vi "Create Master Instance (Serial).vi"(4 "flow control (None)":u16(ring) items=["None", "XON/XOFF", "RTS/CTS", "XON/XOFF & RTS/CTS", "DTR/DSR", "XON/XOFF & DTR/DSR"], 5 "serial type":enum16{"RTU", "ASCII"}(ring), 6 "parity (Even)":u16(ring)=2 items=["None", "Odd", "Even"], 7 "unit ID":u8=1, 8 "error in (no error)":errorcluster, 10 "baud rate (9600)":u32=9600, 11 "VISA resource name":refnum<visa-resource-name>) -> (0 "error out":errorcluster, 3 "serial master instance":refnum<class "Modbus Master.lvclass">)   [LabVIEW 2015, in "Modbus Master.lvclass"]
doc: "Creates a serial or TCP Modbus master instance. You must manually select the polymorphic instance to use."
uses:
  <vilib>/Modbus/master/Modbus Master.lvclass
  <vilib>/Modbus/subvis/Transmission Data Unit (ADU)/RTU Data Unit/RTU Data Unit.lvclass
  <vilib>/Modbus/subvis/Transmission Data Unit (ADU)/ASCII Data Unit/ASCII Data Unit.lvclass
  <vilib>/Modbus/subvis/Transmission Data Unit (ADU)/Transmission Data Unit/Transmission Data Unit.lvclass/Transmission Data Unit.ctl
  <vilib>/Modbus/subvis/Protocol/Serial/Serial Master/Serial Master.lvclass
  <vilib>/Modbus/subvis/Protocol/Serial/Serial Master/Serial Master.lvclass/Serial Master.ctl
  <vilib>/Modbus/master/Modbus Master.lvclass/Modbus Master.ctl
  <vilib>/Modbus/subvis/Modbus API/Modbus API.lvclass/Modbus API.ctl
  <vilib>/Modbus/subvis/Protocol/Serial/Serial Master/Data Access/Serial Data Unit/Write Serial Data Unit.vi
  <vilib>/Modbus/subvis/Protocol/Serial/Serial Master/Data Access/Baud Rate/Write Baud Rate.vi
  <vilib>/Modbus/subvis/Protocol/Serial/Serial Master/Data Access/Parity/Write Parity.vi
  <vilib>/Modbus/subvis/Protocol/Serial/Serial Master/Data Access/VISA resource name/Write VISA resource name.vi
  <vilib>/Modbus/subvis/Protocol/Serial/Serial Master/Data Access/Flow Control/Write Flow Control.vi
  <vilib>/Modbus/subvis/Modbus API/Modbus API.lvclass
  <vilib>/Modbus/subvis/Transmission Data Unit (ADU)/Transmission Data Unit/Transmission Data Unit.lvclass
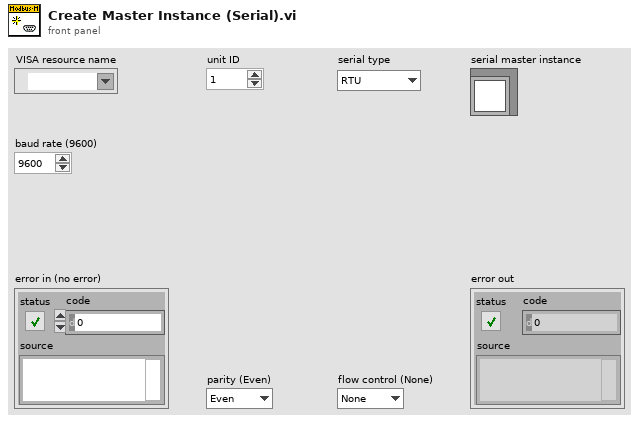
[diagram p1: front panel]
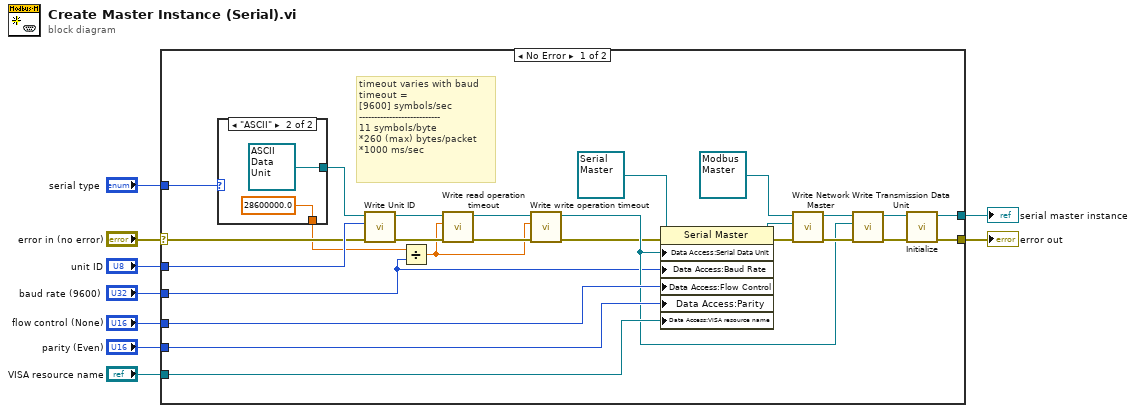
[diagram p0: block diagram]
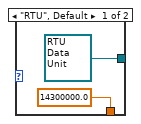
[diagram p2: hidden frame]
diagram:
  n1 = case shown="No Error" "error in (no error)" {
    selector: "error in (no error)" -> [w20 w40]
    tunnel: [w35 w40] -> w9
    tunnel: [w34 _] -> w8
    tunnel: "VISA resource name" -> [w32 _]
    tunnel: "baud rate (9600)" -> [w12 _]
    tunnel: "parity (Even)" -> [w31 _]
    tunnel: "flow control (None)" -> [w30 _]
    tunnel: "serial type" -> [w29 _]
    tunnel: "unit ID" -> [w22 _]
    frame No Error {
      # "timeout varies with baud\ntimeout =\n[9600] symbols/sec\n---------------------------\n11 symbols/byte\n*260 (max) bytes/packet\n*1000 ms/sec"
      n2 = case shown="\"ASCII\"" w29 {
        tunnel: [refnum<class "RTU Data Unit.lvclass"> refnum ("RTU Data Unit") refnum<class "ASCII Data Unit.lvclass"> refnum ("ASCII Data Unit")] -> w23
        tunnel: [14300000.0 ("x") 28600000.0 ("x")] -> w10
        frame "RTU", Default {
        }
        frame "ASCII" {
        }
      }
      n3 = call <vilib>:"Write Unit ID.vi"("error in (no error)"=w20, "unit ID"=w22, "transmission data unit in"=w23) -> ("error out"=w13:errorcluster, "transmission data unit out"=w21:refnum<class "Serial Data Unit.lvclass">)  [unwired: 7 in]
      n4 = Divide(x=w10, y=w12) -> (x/y=w11:dbl)
      n5 = call <vilib>:"Write read operation timeout.vi"("error in (no error)"=w13, "read operation timeout"=w11, "transmission data unit in"=w21) -> ("error out"=w14:errorcluster, "transmission data unit out"=w17:refnum<class "Serial Data Unit.lvclass">)  [unwired: 7 in]
      n6 = call <vilib>:"Write write operation timeout.vi"("error in (no error)"=w14, "write operation timeout"=w11, "transmission data unit in"=w17) -> ("error out"=w15:errorcluster, "transmission data unit out"=w16:refnum<class "Serial Data Unit.lvclass">)  [unwired: 7 in]
      n7 = property class="Serial Master"(reference=refnum<class "Serial Master.lvclass"> refnum ("Serial Master"), error in=w15, "Data Access:Serial Data Unit"=w16, "Data Access:Baud Rate"=w12, "Data Access:Flow Control"=w30, "Data Access:Parity"=w31, "Data Access:VISA resource name"=w32) -> (reference out=w24:refnum<class "Serial Master.lvclass">, error out=w28:errorcluster)
      n8 = call <vilib>:"Write Network Master.vi"("error in (no error)"=w28, "network master"=w24, "Modbus master in"=refnum<class "Modbus Master.lvclass"> refnum ("Modbus Master")) -> ("error out"=w18:errorcluster, "Modbus master out"=w19:refnum<class "Modbus Master.lvclass">)  [unwired: 7 in]
      n9 = call <vilib>:"Write Transmission Data Unit.vi"("error in (no error)"=w18, "transmission data unit"=w16, "Modbus instance in"=w19) -> ("error out"=w25:errorcluster, "Modbus instance out"=w26:refnum<class "Modbus Master.lvclass">)  [unwired: 7 in]
      n10 = call-dynamic "Initialize.vi"("error in (no error)"=w25, "Modbus master in"=w26) -> ("error out"=w35:errorcluster, "Modbus master out"=w34:refnum<class "Modbus Master.lvclass">)  [unwired: 8 in]
    }
    frame Error {
    }
  }
  "error out" <- w9
  "serial master instance" <- w8
